vi "matlab2.vi"   [LabVIEW 2012]
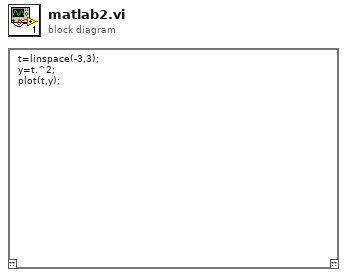
[diagram p0: block diagram]
diagram:
  n1 = script code="t=linspace(-3,3);\ny=t.^2;\nplot(t,y);"() -> ()  [unwired: 1 in, 1 out]
